vi "source_target_converter.vi"(0 "Source High":dbl format="%#_13g", 1 "Source Low":dbl format="%#_13g", 2 "Source":dbl[](array[numeric]) format="%#_13g", 3 "Target Low":dbl format="%#_13g", 4 "Target High":dbl format="%#_13g") -> (5 "Target":dbl[](array[numeric]) format="%#_13g")   [LabVIEW 2016, in "sensor_translation.lvlib"]
uses:
  sensor_translation.lvlib
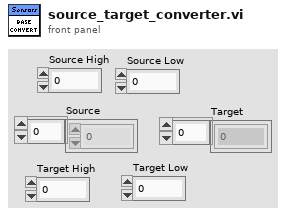
[diagram p1: front panel]
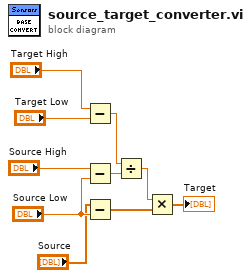
[diagram p0: block diagram]
diagram:
  n1 = Subtract(x="Target High", y="Target Low") -> (x-y=w7:dbl)
  n2 = Subtract(x="Source High", y="Source Low") -> (x-y=w6:dbl)
  n3 = Subtract(x="Source", y="Source Low") -> (x-y=w2:dbl[])
  n4 = Divide(x=w7, y=w6) -> (x/y=w3:dbl)
  n5 = Multiply(x=w3, y=w2) -> (x*y=→"Target":dbl[])
